vi "Version To Tree.vi"(7 "Owning Tree":string, 8 "error in":errorcluster, 11 "Tree Manager in":T1) -> (0 "error out":errorcluster, 3 "Tree Manager out":T1)   [LabVIEW 2020]
uses:
  <vilib>/addons/analyzer/VIAnCFGDataStructure/Tree Manager/Typedefs/Session Handle.ctl
  <vilib>/addons/analyzer/VIAnCFGDataStructure/Tree Manager/Tree.lvclass
  <vilib>/addons/analyzer/VIAnCFGDataStructure/Data Types/Int/Int.lvclass/Int.ctl
  <vilib>/addons/analyzer/VIAnCFGDataStructure/Data Types/Int/To Integer Tree Data.vi
  <vilib>/addons/analyzer/VIAnCFGDataStructure/Data Types/Int/Int.lvclass
  e:/builds/penguin/labview/branches/2020/dev/dist/vi.lib/addons/analyzer/VIAnCFGDataStructure/Tree Data/Tree Data.lvclass
  <vilib>/addons/analyzer/_vianuishared.llb/VIAnUI CFG File Info Global.vi
  <vilib>/addons/analyzer/VIAnCFGDataStructure/Tree Manager/API/Set Attribute Tree Data.vi
  e:/builds/penguin/labview/branches/2020/dev/dist/vi.lib/addons/analyzer/VIAnCFGDataStructure/Data Types/Int/Int.lvclass
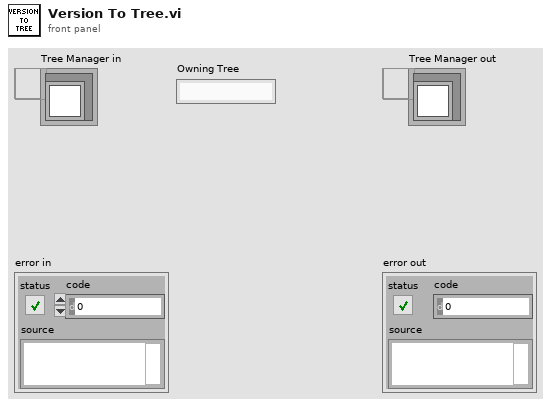
[diagram p1: front panel]
types:
  T1 = typedef "NI_VIAnCFGDataStructure.lvlib/Tree.lvclass/Session Handle.ctl" = refnum<data-value>
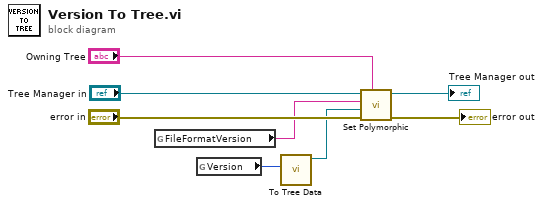
[diagram p0: block diagram]
diagram:
  n1 = global read "VIAnUI CFG File Info Global.vi" "FileFormatVersion"() -> (w3:string)
  n2 = global read "VIAnUI CFG File Info Global.vi" "Version"() -> (w2:i32)
  n3 = call-poly <vilib>:"To Tree Data.vi"("Integer"=w2) -> ("Integer Tree Data"=w6:refnum<class "Int.lvclass">)  [unwired: 10 in]
  n4 = call-poly <vilib>:"Set Polymorphic.vi"("Tree ID"="Owning Tree", "Error In"="error in", "Attribute Value"=w6, "Attribute Name"=w3, "Tree Manager"="Tree Manager in") -> ("Error Out"=→"error out":errorcluster, "Tree Manager"=→"Tree Manager out":T1)  [unwired: 4 in, 1 out]
